vi "Read.vi"(8 "error in (no error)":errorcluster, 11 "ReadoutDevice in":refnum<class "ReadoutDevice.lvclass">) -> (0 "error out":errorcluster, 1 "timed out?":bool=TRUE, 2 "Data":refnum<class "AbstractData.lvclass">, 3 "ReadoutDevice out":refnum<class "ReadoutDevice.lvclass">)   [LabVIEW 2014, in "ReadoutDevice.lvclass"]
uses:
  ReadoutDevice.lvclass
  Model/Data/AbstractData/AbstractData.lvclass
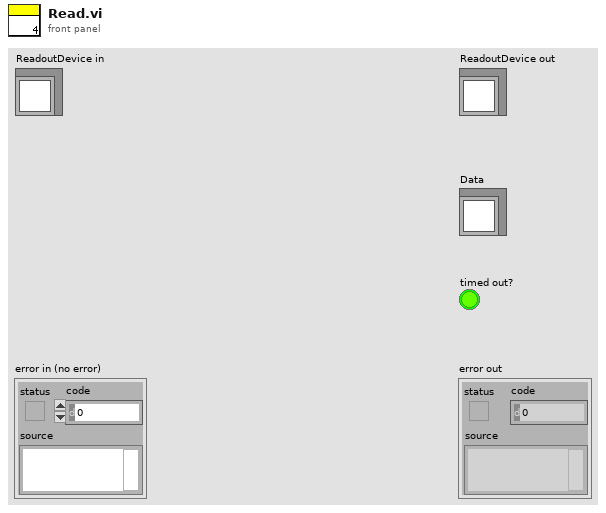
[diagram p1: front panel]
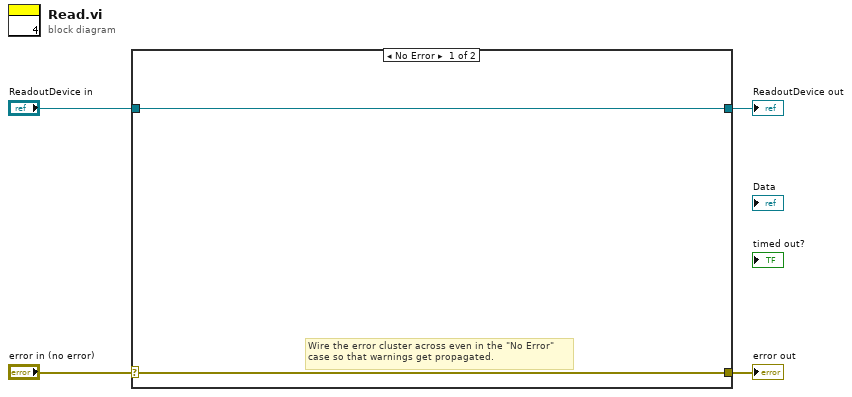
[diagram p0: block diagram]
diagram:
  n1 = case shown="No Error" "error in (no error)" {
    selector: "error in (no error)" -> [w5 w8]
    tunnel: [w5 w8] -> w3
    tunnel: [w6 w7] -> w1
    tunnel: "ReadoutDevice in" -> [w6 w7]
    frame No Error {
      # "Wire the error cluster across even in the \"No Error\"\ncase so that warnings get propagated."
    }
    frame Error {
    }
  }
  "error out" <- w3
  "ReadoutDevice out" <- w1
